vi "BotSpeak_Servo.vi"(0 "Duty (msec)":dbl=1.5, 2 "Bot Settings":T1, 3 "DIO Line":u8(slide) scale=0.0..3.0) -> (1 "response":string="169.254.32.85", 4 "Bot Settings 2":T1)   [LabVIEW 2012]
doc: "Runs a servo motor wired to the specified \"DIO Line\" with the specified \"Duty\" time.\n1 ms is all the way in one direction\n2 ms is all the way in the other direction\n1.5 ms is in the middle"
uses:
  <userlib>/BotSpeak/VIs/Direct/BotSpeak_Control.ctl
panel:
  # "range from 0 to 3 msec"
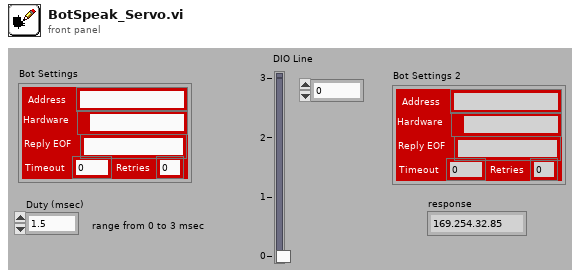
[diagram p1: front panel]
types:
  T1 = typedef "BotSpeak_Control.ctl" = cluster{"Address":string, "Reply EOF":string, "Hardware":path, "Retries":i8, "Timeout":i32}
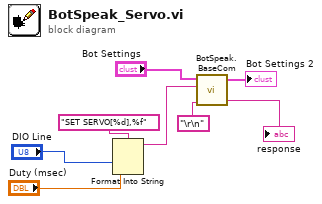
[diagram p0: block diagram]
diagram:
  n1 = Format Into String(format string="SET SERVO[%d],%f" ("command"), "DIO Line", "Duty (msec)") -> (resulting string=w8:string)  [unwired: 2 in, 1 out]
  n2 = call <userlib>:"BotSpeak.BaseCom.vi"("Termination"="\r\n", "command"=w8, "Bot Settings in"="Bot Settings") -> ("response"=→"response":string, "Bot Settings out"=→"Bot Settings 2":T1)  [unwired: 2 in]
